vi "Add_Constant_Speed_Movement_Job.vi"(7 "New Job":bool=TRUE, 8 "error in (no error)":errorcluster, 9 "Tag Item":string, 10 "RotateOrTorqueConstantConfig":T1, 11 "TreeControl in":refnum<vi>) -> (0 "error out":errorcluster, 3 "TreeControl out":refnum<vi>)   [LabVIEW 2021]
uses:
  TypeDefs/RotateOrTorqueConstantConfiguration.ctl
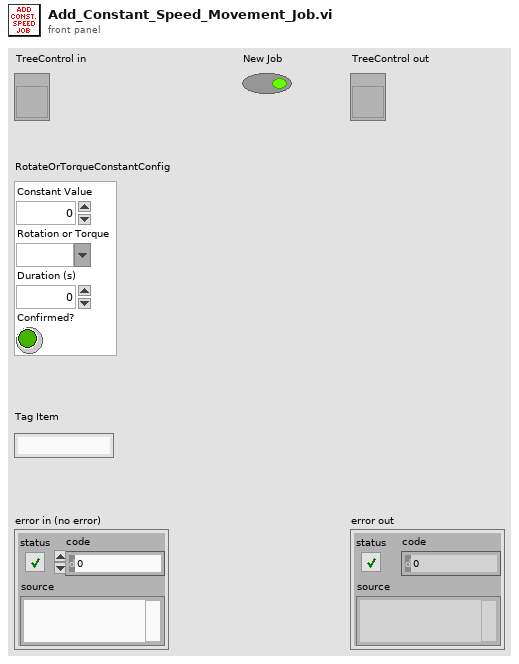
[diagram p1: front panel]
types:
  T1 = typedef "RotateOrTorqueConstantConfiguration.ctl" = cluster{"Constant Value":dbl, "Rotation or Torque":string, "Duration":dbl, "Confirmed?":bool}
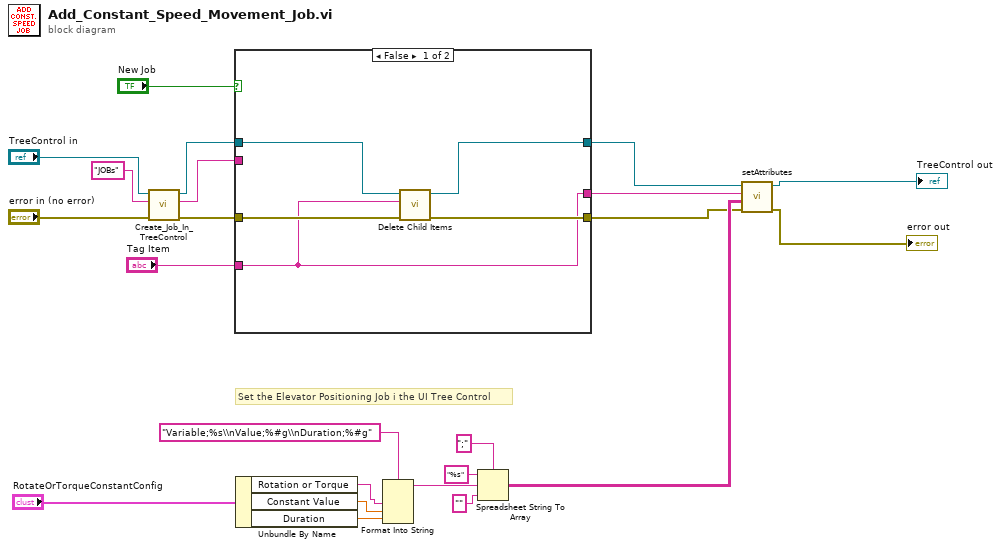
[diagram p0: block diagram]
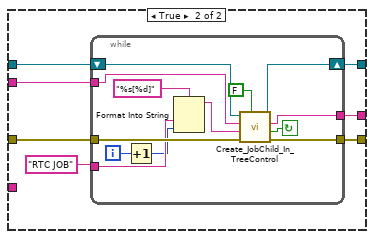
[diagram p2: hidden frame]
diagram:
  # "Set the Elevator Positioning Job i the UI Tree Control"
  n1 = call "Create_Job_In_TreeControl.vi"("error in (no error)"="error in (no error)", "Left Cell String"="JOBs", "TreeControl in"="TreeControl in") -> ("error out"=w19:errorcluster, "Edit Tree Items:Add Item"=w22:string, "TreeControl out"=w23:refnum<vi>)  [unwired: 6 in]
  n2 = case shown="False" "New Job" {
    tunnel: w23 -> [w27 w35]
    tunnel: w22 -> [_ w34]
    tunnel: w19 -> [w28 w33]
    tunnel: [w24 w32] -> w8
    tunnel: [w26 w31] -> w5
    tunnel: [w25 w30] -> w4
    tunnel: "Tag Item" -> [w24 _]
    frame False {
      n3 = call "Delete Child Items.vi"("error in (no error)"=w28, "Item Edit"=w24, "TreeControl in"=w27) -> ("error out"=w25:errorcluster, "TreeControl out"=w26:refnum<vi>)  [unwired: 7 in]
    }
    frame True {
      n4 = while {
        tunnel: w33 -> [w48]
        tunnel: "RTC JOB" -> [w37]
        tunnel: w34 -> [w45]
        tunnel: [w40] -> w30
        tunnel: [w39] -> w32
        shift-right: [w38] -> w31
        shift-left: w35 -> [w44]
        i -> [w42]
        stop <- w41 continue-if-true
        n5 = Increment(x=w42) -> (x+1=w36:i32)
        n6 = Format Into String(format string="%s[%d]", w37, w36) -> (resulting string=w46:string)  [unwired: 2 in, 1 out]
        n7 = call "Create_JobChild_In_TreeControl.vi"("Child Only?"=FALSE, "error in (no error)"=w48, "Child Tag Name"=w46, "Parent Item"=w45, "TreeControl in"=w44) -> ("error out"=w40:errorcluster, "Tag Already Exists?"=w41:bool, "Edit Tree Items:Add Item 2"=w39:string, "TreeControl out"=w38:refnum<vi>)  [unwired: 3 in]
      }
    }
  }
  n8 = Unbundle By Name("RotateOrTorqueConstantConfig") -> ("Rotation or Torque"=w13:string, "Constant Value"=w14:dbl, "Duration"=w16:dbl)
  n9 = Format Into String(format string="Variable;%s\\nValue;%#g\\nDuration;%#g", w13, w14, w16) -> (resulting string=w12:string)  [unwired: 2 in, 1 out]
  n10 = Spreadsheet String To Array(delimiter (Tab)=";", format string="%s", spreadsheet string=w12, array type (2D Dbl)="" ("format string")) -> (array=w9:string[][])
  n11 = call "setAttributes.vi"("error in (no error)"=w4, "Array"=w9, "Edit Tree Items:Add Item in"=w8, "TreeControl in"=w5) -> ("error out"=→"error out":errorcluster, "TreeControl out"=→"TreeControl out":refnum<vi>)  [unwired: 6 in]
